vi "HRR-SetAngLimit.vi"() -> ()   [LabVIEW 2019]
uses:
  <vilib>/FPGAPlugInAG/myRIO-1900/niLvFpga_Open_myRIO-1900.vi
  <vilib>/rvi/interface/common/dynamic/niFpgaDynamicAddResources.vi
  <vilib>/myRIO/Common/Instrument Driver Framework/Utilities/vis/FPGA Ref Manager.vi
  <vilib>/Utility/error.llb/Error Cluster From Error Code.vi
  <vilib>/myRIO/Common/Instrument Driver Framework/Utilities/vis/Ref Counter.vi
  <vilib>/rvi/interface/common/niFpgaWaitOnOcc.vi
  <vilib>/rvi/interface/nirviOpenFPGA/nirviOpenFPGA.xnode
  FPGA Bitfiles/MyRIOFPGATest_FPGATarget_FPGAMainDefault_pJ5Q7Xj1Ujo.lvbitx
  FPGA Main Default.vi
  <vilib>/rvi/interface/nirviMethod/nirviMethod.xnode
  <vilib>/FPGAPlugInAG/Dynamic/niLvFpga_ConfigureFifo_Dynamic.vi
  <vilib>/rvi/errors/niLvFpgaMergeErrorWithErrorCode.vi
  <vilib>/myRIO/Instrument Drivers/Utilities/Utilities.lvlib
panel:
  in  "Angulo limite anti-horario (max)":u16[](array[numeric])=[1023, 1023, 1023, 1023, 1023, 1023, 1023, 1023]
  out "Actual Depth":u32
  in  "Angulo limite horario (min)":u16[](array[numeric])=[0, 0, 0, 0, 0, 0, 0, 0]
  out "FPGA VI Reference Out":refnum<k20>
  out "error out":errorcluster
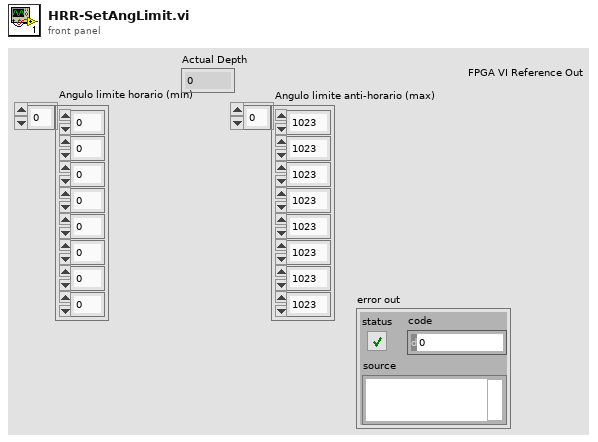
[diagram p1: front panel]
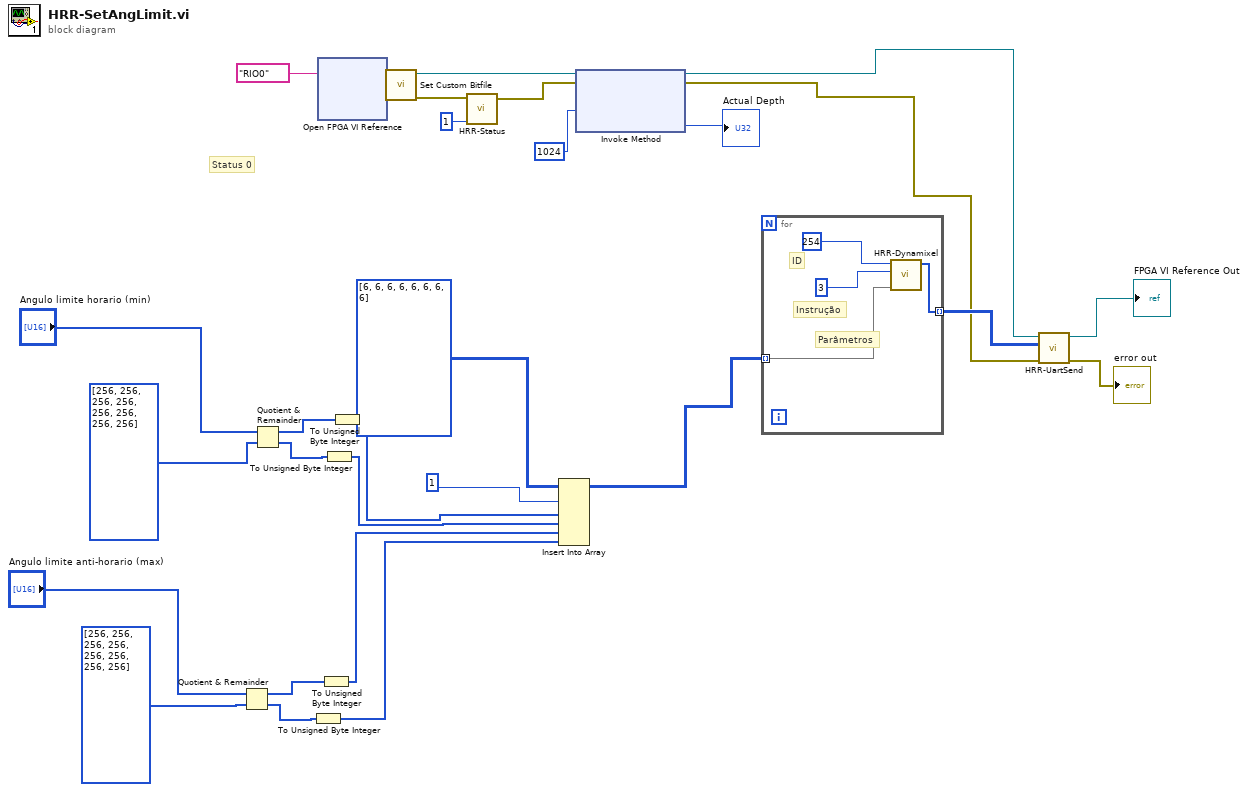
[diagram p0: block diagram]
diagram:
  # "Status 0"
  # "Parâmetros"
  n1 = Quotient & Remainder(x="Angulo limite anti-horario (max)", y=u16[] [256, 256, 256, 256, 256, 256, 256, 256]) -> (x-y*floor(x/y)=w5:u16[], floor(x/y)=w4:u16[])
  n2 = Quotient & Remainder(x="Angulo limite horario (min)", y=u16[] [256, 256, 256, 256, 256, 256, 256, 256]) -> (x-y*floor(x/y)=w11:u16[], floor(x/y)=w10:u16[])
  n3 = To Unsigned Byte Integer(number=w4) -> (unsigned 8bit integer=w1:u8[])
  n4 = xnode "Open FPGA VI Reference"("resource name"=tag "RIO0") -> ("FPGA VI Reference Out"=w21:refnum<k20>, "error out"=w22:errorcluster)  [unwired: 1 in]
  n5 = To Unsigned Byte Integer(number=w5) -> (unsigned 8bit integer=w2:u8[])
  n6 = To Unsigned Byte Integer(number=w10) -> (unsigned 8bit integer=w8:u8[])
  n7 = To Unsigned Byte Integer(number=w11) -> (unsigned 8bit integer=w9:u8[])
  n8 = call <vilib>:"Set Custom Bitfile.vi"("error in (no error)"=w22, "Custom FPGA Reference In"=w21) -> ("error out"=w15:errorcluster, "Custom FPGA Reference Out"=w16:refnum<k20>)  [unwired: 8 in]
  n9 = call "HRR-Status.vi"("Status (U4)"=u8 1 ("number"), "error in (no error)"=w15) -> ("error out"=w18:errorcluster)  [unwired: 9 in]
  n10 = Insert Into Array(array=u8[][] [[6], [6], [6], [6], [6], [6], [6], [6]], index (col)=1 ("disabled index (col)"), new element #1=w9, new element #2=w8, new element #3=w2, new element #4=w1) -> (w27:u8[][])  [unwired: 1 in]
  n11 = xnode "Invoke Method"("FPGA VI Reference In"=w16, "error in"=w18, "Requested Depth"=u32 1024) -> ("FPGA VI Reference Out"=w13:refnum<k20>, "error out"=w14:errorcluster, "Actual Depth"=→"Actual Depth":u32)
  n12 = for {
    tunnel: w27 -> [w31] mode=indexing
    tunnel: [w30] -> w24 mode=indexing
    # "Instrução"
    # "ID"
    n13 = call "HRR-Dynamixel.vi"("ID"=u8 254, "Instruction"=u8 3, "Array in"=w31) -> ("Array out"=w30:u8[])  [unwired: 7 in]
  }
  n14 = call "HRR-UartSend.vi"("error in (no error)"=w14, "Array"=w24, "Refnum in"=w13) -> ("error out"=→"error out":errorcluster, "Refnum out"=→"FPGA VI Reference Out":refnum<k20>)  [unwired: 7 in]
